vi "Get Mode.vi"(8 "error in (no error)":errorcluster, 11 "Camera in":refnum<class "Camera.lvclass">) -> (0 "error out":errorcluster, 2 "State":enum16{"Idle", "Live Mode", "Streaming"}(ring), 3 "Camera out":refnum<class "Camera.lvclass">)   [LabVIEW 2023, in "Camera.lvlib" / "Camera.lvclass"]
uses:
  Camera.lvclass
  Camera.lvclass/Camera.ctl
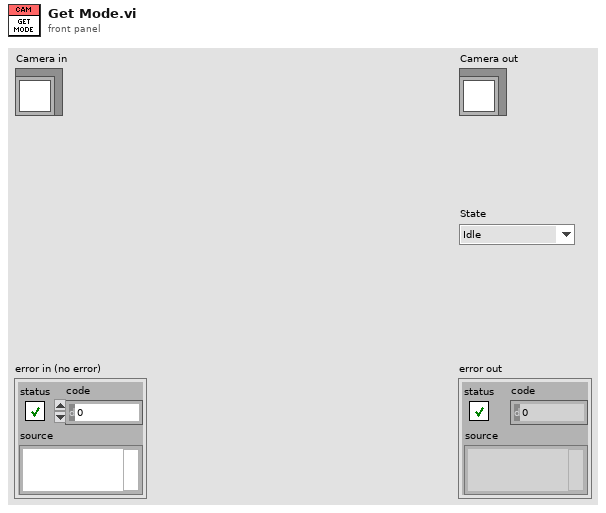
[diagram p1: front panel]
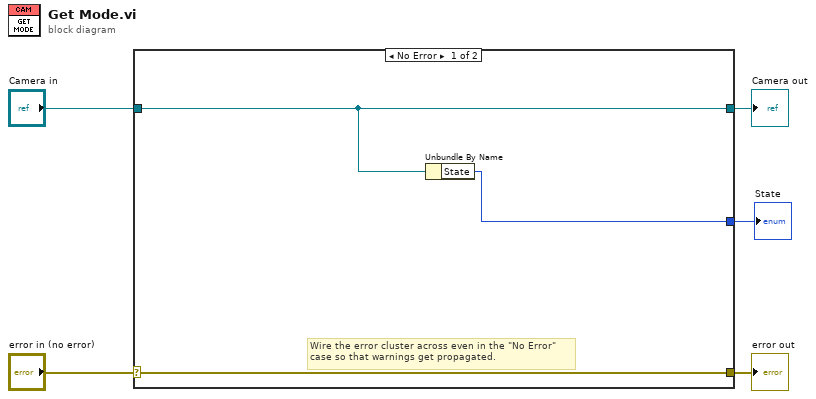
[diagram p0: block diagram]
diagram:
  n1 = case shown="No Error" "error in (no error)" {
    selector: "error in (no error)" -> [w8 w10]
    tunnel: [w8 w10] -> w4
    tunnel: [w7 w9] -> w2
    tunnel: "Camera in" -> [w7 w9]
    tunnel: [w6 _] -> w1
    frame No Error {
      # "Wire the error cluster across even in the \"No Error\"\ncase so that warnings get propagated."
      n2 = Unbundle By Name(w7) -> ("State"=w6:enum16{"Idle", "Live Mode", "Streaming"})
    }
    frame Error {
    }
  }
  "error out" <- w4
  "Camera out" <- w2
  "State" <- w1
